vi "quiz3.1.vi"() -> ()   [LabVIEW 2017]
uses:
  <vilib>/Utility/file.llb/Read Delimited Spreadsheet (string).vi
panel:
  out "Tab Control 2":T1(tab)
  in  "Contraseña 2":string
  in  "Login 2":string
  in  "Ingresar 2":bool=TRUE
  in  "Ingrese posicion 2":i32
  in  "Usuario a borrar 2":string
  in  "Agregar 2":bool
  in  "Nuevo usuario 2":string
  in  "Nueva contraseña 2":string
  in  "eliminar 2":bool
  in  "Terminar sesion 3":bool
  out "Usuario 2":string
  in  "Terminar sesion 4":bool
  out "leeradd 2":string[][](array[string])
  out "element 4":string
  out "Usuarios y contraseñas 2":string[](array[string])
  out "element 3":i32
  out "Usuarios 2":string[](array[string])
  out "Usuarios":string[](array[string])
  out "element 2":i32
  out "Usuarios y contraseñas":string[](array[string])
  out "leeradd":string[][](array[string])
  out "element":string
  out "Tab Control":T1(tab)
  in  "Contraseña":string
  in  "Login":string
  in  "Ingresar":bool=TRUE
  in  "Ingrese posicion":i32
  in  "Usuario a borrar":string
  in  "Agregar":bool
  in  "Nuevo usuario":string
  in  "Nueva contraseña":string
  in  "eliminar":bool
  in  "Terminar sesion 2":bool
  out "Usuario":string
  in  "Terminar sesion":bool
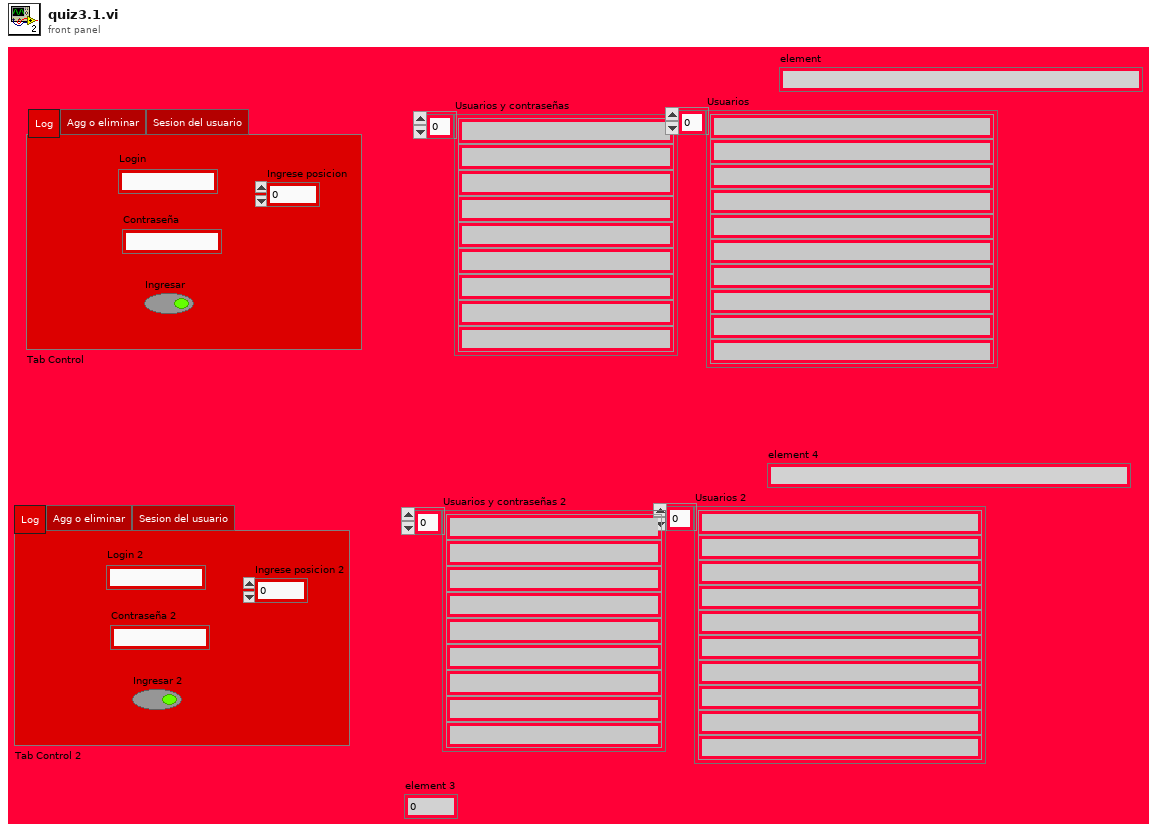
[diagram p1: front panel]
types:
  T1 = enum32{"Log", "Agg o eliminar", "Sesion del usuario"}
  T2 = enum16{"open", "replace", "create", "open or create", "replace or create", "replace or create with confirmation"}
  T3 = typedef "Semaphore RefNum" = refnum<k1>
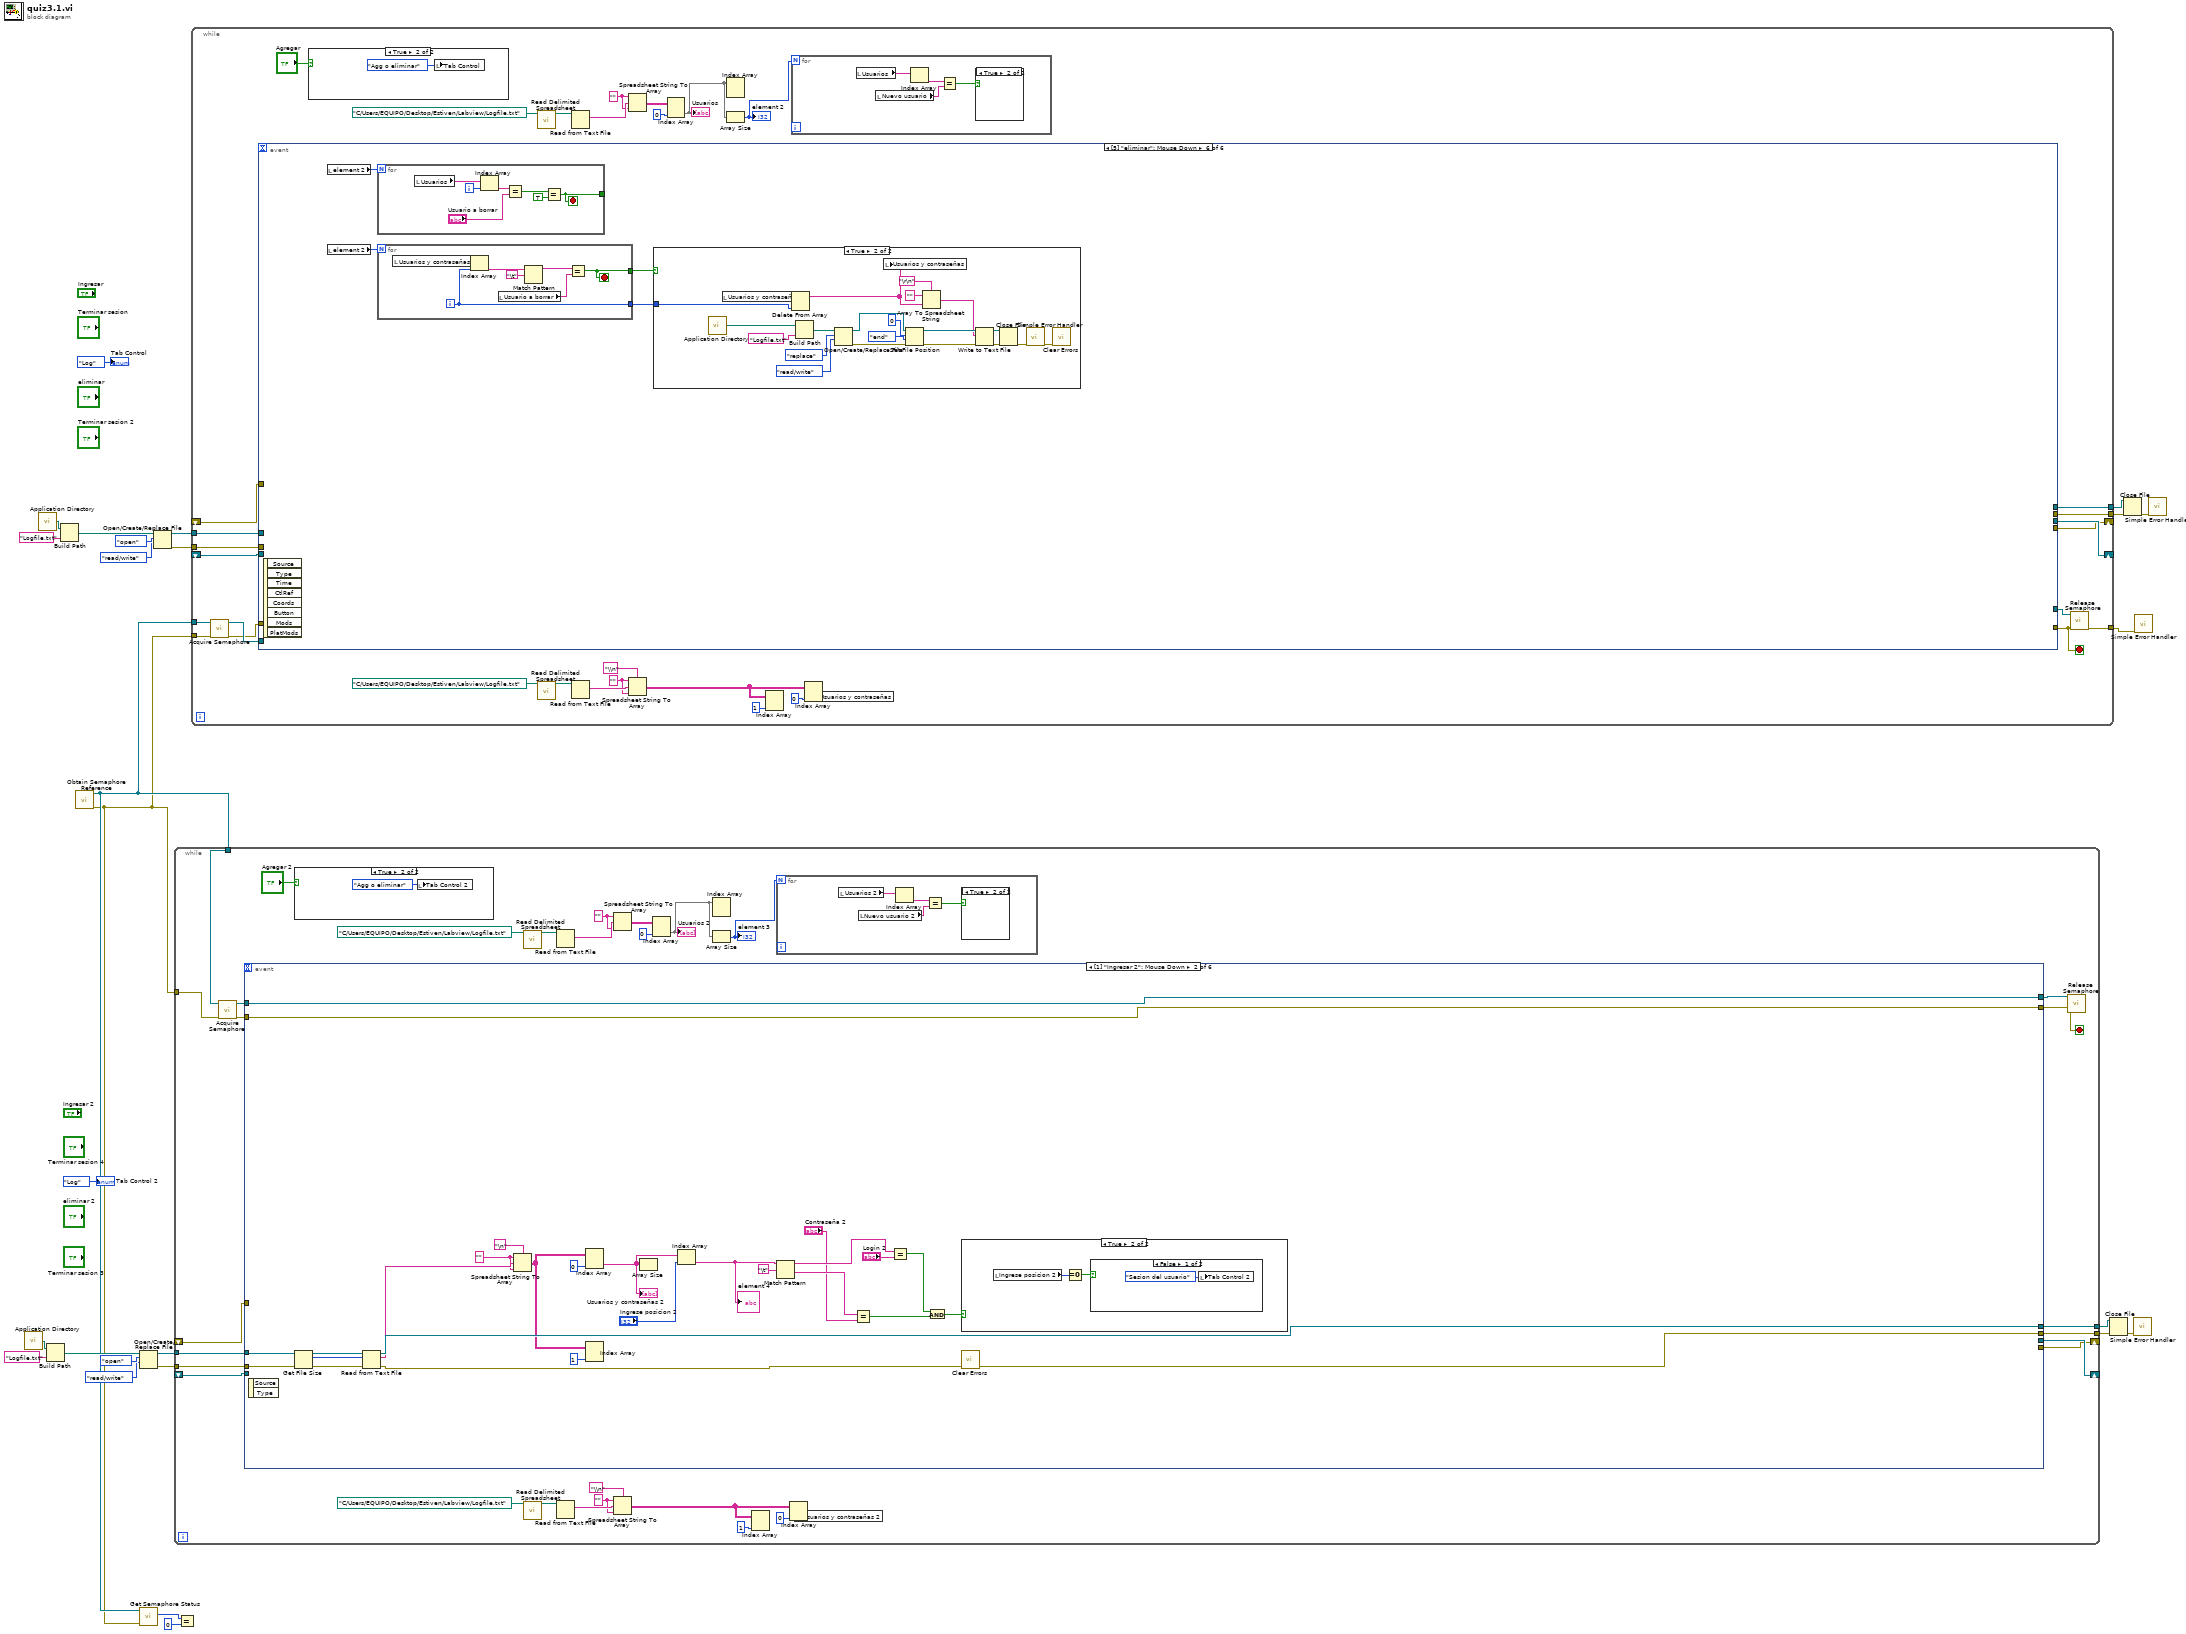
[diagram p0: block diagram]
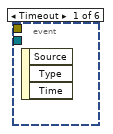
[diagram p4: hidden frame]
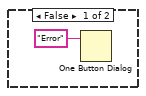
[diagram p5: hidden frame]
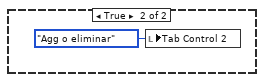
[diagram p6: hidden frame]
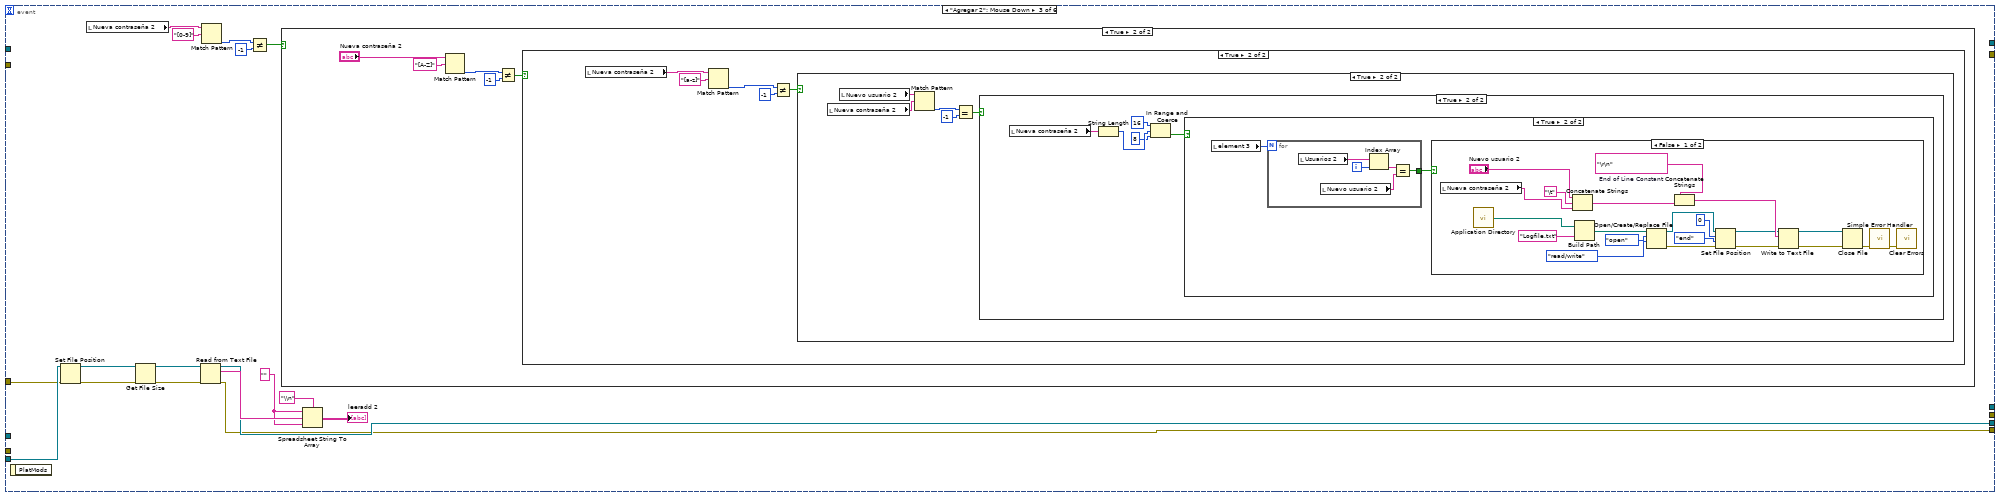
[diagram p7: hidden frame]
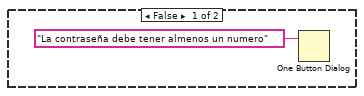
[diagram p8: hidden frame]
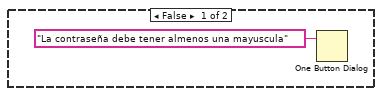
[diagram p9: hidden frame]
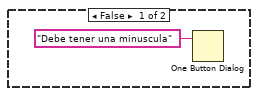
[diagram p10: hidden frame]
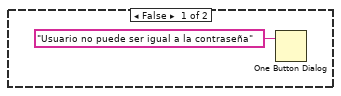
[diagram p11: hidden frame]
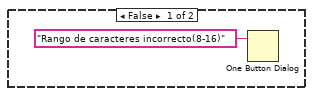
[diagram p12: hidden frame]
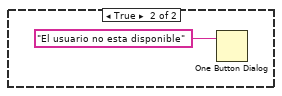
[diagram p13: hidden frame]
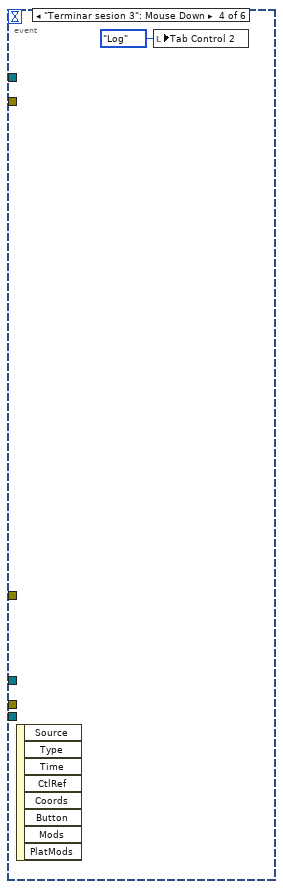
[diagram p14: hidden frame]
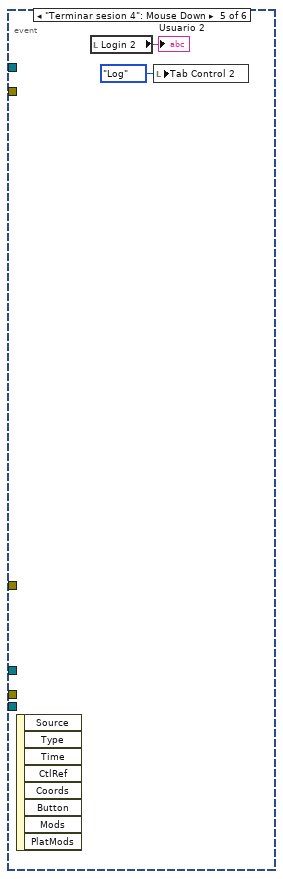
[diagram p15: hidden frame]
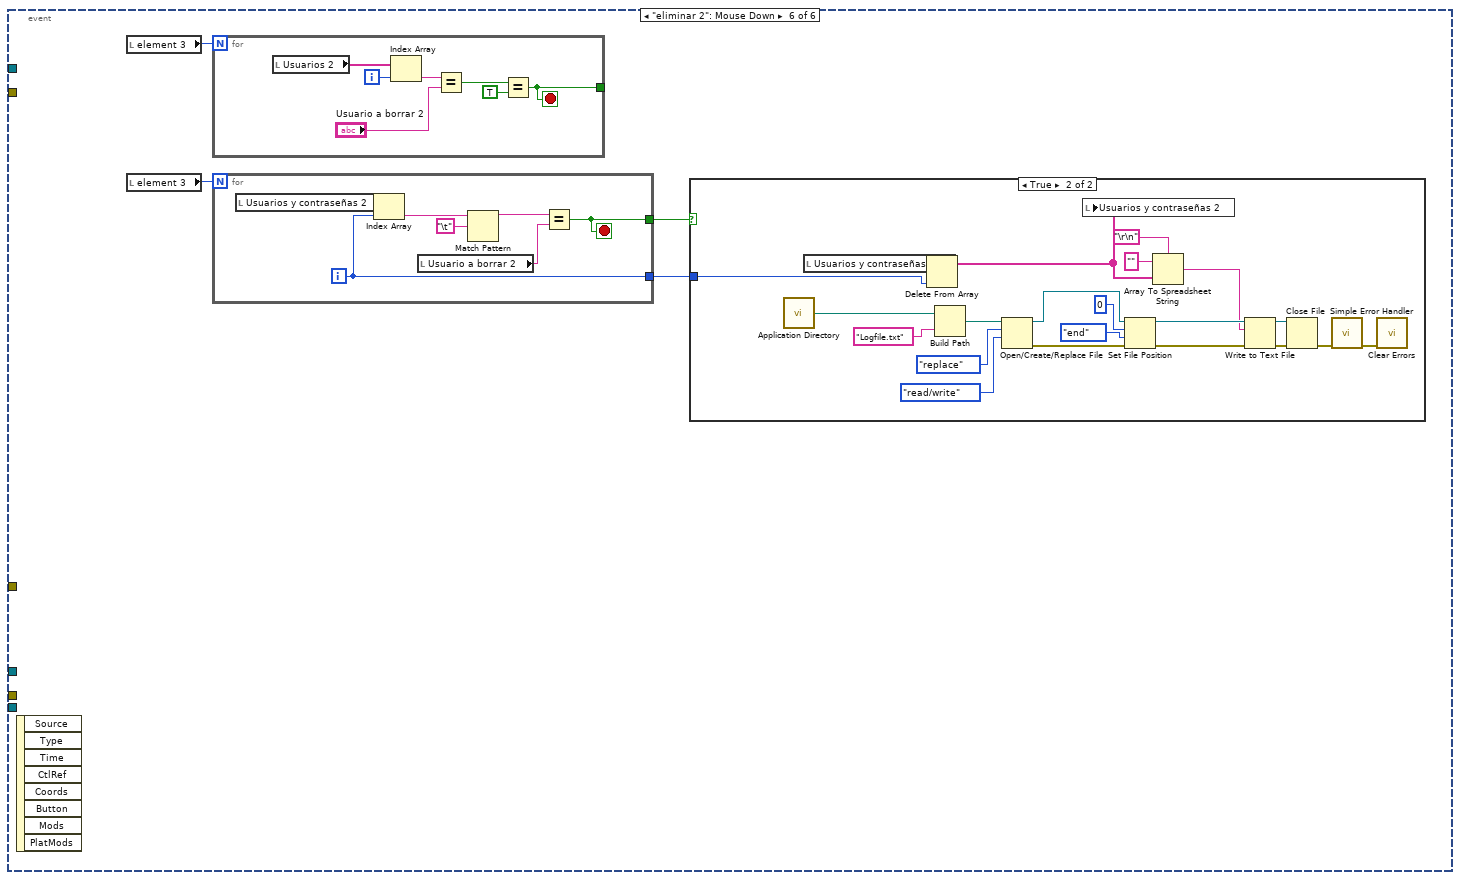
[diagram p16: hidden frame]
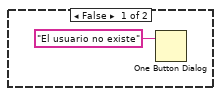
[diagram p17: hidden frame]
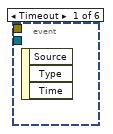
[diagram p20: hidden frame]
diagram:
  n1 = call <vilib>:"Application Directory.vi"() -> ("Application Directory"=w10:path)
  n2 = call <vilib>:"Application Directory.vi"() -> ("Application Directory"=w21:path)
  n3 = Build Path(base path=w10, name or relative path="Logfile.txt") -> (appended path=w11:path)
  n4 = Build Path(base path=w21, name or relative path="Logfile.txt") -> (appended path=w22:path)
  n5 = call <vilib>:"Obtain Semaphore Reference.vi"() -> ("error out"=w3:errorcluster, "semaphore"=w4:T3)  [unwired: 5 in, 1 out]
  n6 = Open/Create/Replace File(file path (use dialog)=w11, operation (0:open)=T2."open", access (0:read/write)=enum16{"read/write", "read-only", "write-only"}."read/write") -> (refnum out=w13:refnum<file>, error out=w16:errorcluster)  [unwired: 3 in, 1 out]
  n7 = call <vilib>:"Get Semaphore Status.vi"("error in (no error)"=w3, "semaphore"=w4) -> ("# available"=w2:i32)  [unwired: 4 in, 5 out]
  n8 = Open/Create/Replace File(file path (use dialog)=w22, operation (0:open)=T2."open", access (0:read/write)=enum16{"read/write", "read-only", "write-only"}."read/write") -> (refnum out=w24:refnum<file>, error out=w27:errorcluster)  [unwired: 3 in, 1 out]
  n9 = while {
    tunnel: w16 -> [w55]
    tunnel: [w59] -> w15
    tunnel: w13 -> [w58]
    tunnel: [w57] -> w12
    shift-right: [w52] -> _
    shift-left: _ -> [w54]
    shift-right: [w51] -> _
    shift-left: _ -> [w53]
    tunnel: w4 -> [w33]
    tunnel: w3 -> [w32]
    stop <- w28 stop-if-true
    w36 = "" ("format string")
    w46 = "" ("format string")
    n10 = call <vilib>:"Acquire Semaphore.vi"("error in (no error)"=w32, "semaphore"=w33) -> ("error out"=w29:errorcluster, "semaphore out"=w31:T3)  [unwired: 3 in, 1 out]
    n11 = event shown="[1] \"Ingresar 2\": Mouse Down" {
      selector: _ -> [_ _ _ _ _ _]
      dyn-events: _ -> [_ _ _ _ _ _]
      timeout: _ -> [_ _ _ _ _ _]
      tunnel: w55 -> [_ w83 _ _ _ _]
      tunnel: [_ w90 _ _ _ _] -> w59
      tunnel: w58 -> [_ w84 _ _ _ _]
      tunnel: [_ w86 _ _ _ _] -> w57
      tunnel: w54 -> [_ _ w101 _ _ _]
      tunnel: w53 -> [_ _ w100 _ _ _]
      tunnel: [_ _ w98 _ _ _] -> w52
      tunnel: [_ _ w97 _ _ _] -> w51
      tunnel: [_ w66 _ _ _ _] -> w30
      tunnel: w31 -> [_ w66 _ _ _ _]
      tunnel: w29 -> [_ w65 _ _ _ _]
      tunnel: [_ w65 _ _ _ _] -> w28
      event Timeout {
        n12 = event-data() -> ()  [unwired: 1 in, 3 out]
      }
      event "Ingresar 2": Mouse Down {
        w76 = "" ("format string")
        n13 = event-data() -> ()  [unwired: 1 in, 2 out]
        n14 = Get File Size(file=w84, error in=w83) -> (refnum out=w82:refnum<file>, size (in bytes)=w81:i64, 0:w80:errorcluster)
        n15 = Read from Text File(file (use dialog)=w82, count=w81, error in=w80) -> (refnum out=w86:refnum<file>, text=w77:string, error out=w91:errorcluster)  [unwired: 1 in, 1 out]
        n16 = Spreadsheet String To Array(delimiter (Tab)="\n", format string=w76, spreadsheet string=w77, array type (2D Dbl)=w76) -> (array=w75:string[][])
        n17 = Index Array "Index Array"(array=w75, index (col)=0 ("disabled index (col)")) -> (element=w67:string[])  [unwired: 1 in]
        "Usuarios y contraseñas 2" <- w67
        n18 = Index Array "Index Array"(array=w75, index (col)=1 ("disabled index (col)")) -> ()  [unwired: 1 in, 1 out]
        n19 = Array Size(array=w67) -> ()  [unwired: 1 out]
        n20 = Index Array "Index Array"(array=w67, index="Ingrese posicion 2") -> (element=w68:string)
        "element 4" <- w68
        n21 = Match Pattern(string=w68, regular expression="\t") -> (before substring=w79:string, after substring=w78:string)  [unwired: 1 in, 2 out]
        n22 = Equal?(x=w78, y="Contraseña 2") -> (x = y?=w88:bool)
        n23 = Equal?(x=w79, y="Login 2") -> (x = y?=w89:bool)
        n24 = And(x=w89, y=w88) -> (x .and. y?=w87:bool)
        n25 = case shown="True" w87 {
          frame False {
            n26 = One Button Dialog(message="Error") -> ()  [unwired: 1 in, 1 out]
          }
          frame True {
            n27 = local read "Ingrese posicion 2"() -> (w94:i32)
            n28 = Equal To 0?(x=w94) -> (x = 0?=w93:bool)
            n29 = case shown="False" w93 {
              frame False {
                n30 = local write "Tab Control 2"(T1."Sesion del usuario" ("Tab Control")) -> ()
              }
              frame True {
                n31 = local write "Tab Control 2"(enum32{"Log", "Agg o eliminar"}."Agg o eliminar" ("Tab Control")) -> ()
              }
            }
          }
        }
        n32 = call <vilib>:"Clear Errors.vi"("error in (no error)"=w91) -> ("error out"=w90:errorcluster)  [unwired: 5 in, 1 out]
      }
      event "Agregar 2": Mouse Down {
        w102 = "" ("format string")
        n33 = event-data() -> ()  [unwired: 1 in, 1 out]
        n34 = Set File Position(refnum=w101, error in=w100) -> (refnum out=w108:refnum<file>, error out=w105:errorcluster)  [unwired: 2 in]
        n35 = local read "Nueva contraseña 2"() -> (w113:string)
        n36 = Get File Size(file=w108, error in=w105) -> (refnum out=w107:refnum<file>, 0:w104:errorcluster)  [unwired: 1 out]
        n37 = Read from Text File(file (use dialog)=w107, error in=w104) -> (refnum out=w98:refnum<file>, text=w106:string, error out=w97:errorcluster)  [unwired: 2 in, 1 out]
        n38 = Match Pattern(string=w113, regular expression="[0-9]") -> (offset past match=w111:i32)  [unwired: 1 in, 3 out]
        n39 = Not Equal?(x=w111, y=-1) -> (x != y?=w109:bool)
        n40 = case shown="True" w109 {
          frame False {
            n41 = One Button Dialog(message="La contraseña debe tener almenos un numero") -> ()  [unwired: 1 in, 1 out]
          }
          frame True {
            n42 = Match Pattern(string="Nueva contraseña 2", regular expression="[A-Z]") -> (offset past match=w118:i32)  [unwired: 1 in, 3 out]
            n43 = Not Equal?(x=w118, y=-1) -> (x != y?=w115:bool)
            n44 = case shown="True" w115 {
              frame False {
                n45 = One Button Dialog(message="La contraseña debe tener almenos una mayuscula") -> ()  [unwired: 1 in, 1 out]
              }
              frame True {
                n46 = local read "Nueva contraseña 2"() -> (w122:string)
                n47 = Match Pattern(string=w122, regular expression="[a-z]") -> (offset past match=w124:i32)  [unwired: 1 in, 3 out]
                n48 = Not Equal?(x=w124, y=-1) -> (x != y?=w121:bool)
                n49 = case shown="True" w121 {
                  frame False {
                    n50 = One Button Dialog(message="Debe tener una minuscula") -> ()  [unwired: 1 in, 1 out]
                  }
                  frame True {
                    n51 = local read "Nueva contraseña 2"() -> (w131:string)
                    n52 = local read "Nuevo usuario 2"() -> (w130:string)
                    n53 = Match Pattern(string=w130, regular expression=w131) -> (offset past match=w129:i32)  [unwired: 1 in, 3 out]
                    n54 = Equal?(x=w129, y=-1) -> (x = y?=w128:bool)
                    n55 = case shown="True" w128 {
                      frame False {
                        n56 = One Button Dialog(message="Usuario no puede ser igual a la contraseña") -> ()  [unwired: 1 in, 1 out]
                      }
                      frame True {
                        n57 = local read "Nueva contraseña 2"() -> (w137:string)
                        n58 = String Length(string=w137) -> (length=w136:i32)
                        n59 = In Range and Coerce(upper limit=16, x=w136, lower limit=8) -> (In Range?=w133:bool)  [unwired: 1 out]
                        n60 = case shown="True" w133 {
                          frame False {
                            n61 = One Button Dialog(message="Rango de caracteres incorrecto(8-16)") -> ()  [unwired: 1 in, 1 out]
                          }
                          frame True {
                            n62 = local read "element 3"() -> (w140:i32)
                            n63 = for {
                              N: w140 -> [_]
                              tunnel: [w165] -> w139
                              i -> [w163]
                              n64 = local read "Usuarios 2"() -> (w164:string[])
                              n65 = local read "Nuevo usuario 2"() -> (w167:string)
                              n66 = Index Array(array=w164, index=w163) -> (element=w166:string)
                              n67 = Equal?(x=w166, y=w167) -> (x = y?=w165:bool)
                            }
                            n68 = case shown="False" w139 {
                              frame False {
                                w147 = "\r\n"  # End of Line Constant
                                n69 = local read "Nueva contraseña 2"() -> (w148:string)
                                n70 = call <vilib>:"Application Directory.vi"() -> ("Application Directory"=w150:path)
                                n71 = Concatenate Strings "Concatenate Strings"("Nuevo usuario 2", "\t", w148) -> (w161:string)
                                n72 = Build Path(base path=w150, name or relative path="Logfile.txt") -> (appended path=w151:path)
                                n73 = Open/Create/Replace File(file path (use dialog)=w151, operation (0:open)=T2."open", access (0:read/write)=enum16{"read/write", "read-only", "write-only"}."read/write") -> (refnum out=w152:refnum<file>, error out=w155:errorcluster)  [unwired: 3 in, 1 out]
                                n74 = Concatenate Strings "Concatenate Strings"(w147, w161) -> (w160:string)
                                n75 = Set File Position(offset (in bytes) (0)=i64 0, refnum=w152, from (0:start)=enum16{"start", "end", "current"}."end", error in=w155) -> (refnum out=w153:refnum<file>, error out=w156:errorcluster)
                                n76 = Write to Text File(file (use dialog)=w153, text=w160, error in=w156) -> (refnum out=w154:refnum<file>, error out=w157:errorcluster)  [unwired: 1 in, 1 out]
                                n77 = Close File(refnum=w154, error in=w157) -> (error out=w158:errorcluster)  [unwired: 1 out]
                                n78 = call <vilib>:"Simple Error Handler.vi"("error in (no error)"=w158) -> ("error out"=w159:errorcluster)  [unwired: 4 in, 4 out]
                                n79 = call <vilib>:"Clear Errors.vi"("error in (no error)"=w159) -> ()  [unwired: 5 in, 2 out]
                              }
                              frame True {
                                n80 = One Button Dialog(message="El usuario no esta disponible") -> ()  [unwired: 1 in, 1 out]
                              }
                            }
                          }
                        }
                      }
                    }
                  }
                }
              }
            }
          }
        }
        n81 = Spreadsheet String To Array(delimiter (Tab)="\\n", format string=w102, spreadsheet string=w106, array type (2D Dbl)=w102) -> (array=→"leeradd 2":string[][])
      }
      event "Terminar sesion 3": Mouse Down {
        n82 = event-data() -> ()  [unwired: 1 in, 8 out]
        n83 = local write "Tab Control 2"(T1."Log" ("Tab Control")) -> ()
      }
      event "Terminar sesion 4": Mouse Down {
        n84 = event-data() -> ()  [unwired: 1 in, 8 out]
        n85 = local read "Login 2"() -> (→"Usuario 2":string)
        n86 = local write "Tab Control 2"(T1."Log" ("Tab Control")) -> ()
      }
      event "eliminar 2": Mouse Down {
        n87 = event-data() -> ()  [unwired: 1 in, 8 out]
        n88 = local read "element 3"() -> (w174:i32)
        n89 = local read "element 3"() -> (w173:i32)
        n90 = for {
          N: w174 -> [_]
          tunnel: [w183] -> _
          i -> [w182]
          stop <- w183 stop-if-true
          n91 = local read "Usuarios 2"() -> (w185:string[])
          n92 = Index Array(array=w185, index=w182) -> (element=w184:string)
          n93 = Equal?(x=w184, y="Usuario a borrar 2") -> (x = y?=w188:bool)
          n94 = Equal?(x=w188, y=TRUE) -> (x = y?=w183:bool)
        }
        n95 = for {
          N: w173 -> [_]
          tunnel: [w177] -> w171
          tunnel: [w175] -> w172
          i -> [w175]
          stop <- w177 stop-if-true
          n96 = local read "Usuarios y contraseñas 2"() -> (w176:string[])
          n97 = Index Array(array=w176, index=w175) -> (element=w181:string)
          n98 = local read "Usuario a borrar 2"() -> (w178:string)
          n99 = Match Pattern(string=w181, regular expression="\t") -> (before substring=w179:string)  [unwired: 1 in, 3 out]
          n100 = Equal?(x=w179, y=w178) -> (x = y?=w177:bool)
        }
        n101 = case shown="True" w171 {
          tunnel: w172 -> [_ w195]
          frame False {
            n102 = One Button Dialog(message="El usuario no existe") -> ()  [unwired: 1 in, 1 out]
          }
          frame True {
            n103 = call <vilib>:"Application Directory.vi"() -> ("Application Directory"=w201:path)
            n104 = local read "Usuarios y contraseñas 2"() -> (w194:string[])
            n105 = Delete From Array "Delete From Array"(array=w194, index=w195) -> (array with subset deleted=w192:string[])  [unwired: 1 in, 1 out]
            n106 = Build Path(base path=w201, name or relative path="Logfile.txt") -> (appended path=w202:path)
            n107 = Open/Create/Replace File(file path (use dialog)=w202, operation (0:open)=T2."replace", access (0:read/write)=enum16{"read/write", "read-only", "write-only"}."read/write") -> (refnum out=w203:refnum<file>, error out=w206:errorcluster)  [unwired: 3 in, 1 out]
            n108 = local write "Usuarios y contraseñas 2"(w192) -> ()
            n109 = Set File Position(offset (in bytes) (0)=i64 0, refnum=w203, from (0:start)=enum16{"start", "end", "current"}."end", error in=w206) -> (refnum out=w204:refnum<file>, error out=w207:errorcluster)
            n110 = Array To Spreadsheet String(delimiter (Tab)="\r\n", array=w192, 3:"" ("format string")) -> (spreadsheet string=w191:string)
            n111 = Write to Text File(file (use dialog)=w204, text=w191, error in=w207) -> (refnum out=w205:refnum<file>, error out=w208:errorcluster)  [unwired: 1 in, 1 out]
            n112 = Close File(refnum=w205, error in=w208) -> (error out=w209:errorcluster)  [unwired: 1 out]
            n113 = call <vilib>:"Simple Error Handler.vi"("error in (no error)"=w209) -> ("error out"=w210:errorcluster)  [unwired: 4 in, 4 out]
            n114 = call <vilib>:"Clear Errors.vi"("error in (no error)"=w210) -> ()  [unwired: 5 in, 2 out]
          }
        }
      }
    }
    n115 = case shown="True" "Agregar 2" {
      frame False {
      }
      frame True {
        n116 = local write "Tab Control 2"(T1."Agg o eliminar" ("Tab Control")) -> ()
      }
    }
    n117 = call-poly <vilib>:"Read Delimited Spreadsheet.vi"("file path (dialog if empty)"=path "C:/Users/EQUIPO/Desktop/Estiven/Labview/Logfile.txt") -> ("new file path (Not A Path if cancelled)"=w47:path)  [unwired: 9 in, 5 out]
    n118 = call-poly <vilib>:"Read Delimited Spreadsheet.vi"("file path (dialog if empty)"=path "C:/Users/EQUIPO/Desktop/Estiven/Labview/Logfile.txt") -> ("new file path (Not A Path if cancelled)"=w42:path)  [unwired: 9 in, 5 out]
    n119 = Read from Text File(file (use dialog)=w47) -> (text=w48:string)  [unwired: 3 in, 3 out]
    n120 = Read from Text File(file (use dialog)=w42) -> (text=w41:string)  [unwired: 3 in, 3 out]
    n121 = Spreadsheet String To Array(format string=w46, spreadsheet string=w48, array type (2D Dbl)=w46) -> (array=w49:string[][])  [unwired: 1 in]
    n122 = Spreadsheet String To Array(delimiter (Tab)="\\n", format string=w36, spreadsheet string=w41, array type (2D Dbl)=w36) -> (array=w40:string[][])
    n123 = Index Array(array=w49, index (col)=0 ("index")) -> (element=w43:string[])  [unwired: 1 in]
    "Usuarios 2" <- w43
    n124 = Index Array "Index Array"(array=w43) -> ()  [unwired: 2 in, 2 out]
    n125 = Array Size(array=w43) -> (size(s)=w50:i32)
    "element 3" <- w50
    n126 = Index Array(array=w40, index (col)=1 ("disabled index (col)")) -> ()  [unwired: 1 in, 1 out]
    n127 = for {
      N: w50 -> [_]
      n128 = local read "Usuarios 2"() -> (w63:string[])
      n129 = local read "Nuevo usuario 2"() -> (w61:string)
      n130 = Index Array(array=w63) -> (element=w62:string)  [unwired: 1 in]
      n131 = Equal?(x=w62, y=w61) -> (x = y?=w60:bool)
      n132 = case shown="True" w60 {
        frame False {
        }
        frame True {
        }
      }
    }
    n133 = Index Array(array=w40, index (col)=0 ("index")) -> (element=w39:string[])  [unwired: 1 in]
    n134 = local write "Usuarios y contraseñas 2"(w39) -> ()
    n135 = call <vilib>:"Release Semaphore.vi"("error in (no error)"=w28, "semaphore"=w30) -> ()  [unwired: 4 in, 2 out]
  }
  n136 = Equal?(x=w2, y=0) -> ()  [unwired: 1 out]
  n137 = while {
    tunnel: w27 -> [w239]
    tunnel: [w243] -> w26
    tunnel: w24 -> [w242]
    tunnel: [w241] -> w23
    shift-right: [w236] -> _
    shift-left: _ -> [w238]
    shift-right: [w235] -> _
    shift-left: _ -> [w237]
    tunnel: w4 -> [w217]
    tunnel: w3 -> [w216]
    tunnel: [w211] -> w5
    stop <- w212 stop-if-true
    w220 = "" ("format string")
    w230 = "" ("format string")
    n138 = call <vilib>:"Acquire Semaphore.vi"("error in (no error)"=w216, "semaphore"=w217) -> ("error out"=w213:errorcluster, "semaphore out"=w215:T3)  [unwired: 3 in, 1 out]
    n139 = event shown="[5] \"eliminar\": Mouse Down" {
      selector: _ -> [_ _ _ _ _ _]
      dyn-events: _ -> [_ _ _ _ _ _]
      timeout: _ -> [_ _ _ _ _ _]
      tunnel: w239 -> [_ w267 _ _ _ _]
      tunnel: [_ w274 _ _ _ _] -> w243
      tunnel: w242 -> [_ w268 _ _ _ _]
      tunnel: [_ w270 _ _ _ _] -> w241
      tunnel: w238 -> [_ _ w286 _ _ _]
      tunnel: w237 -> [_ _ w285 _ _ _]
      tunnel: [_ _ w283 _ _ _] -> w236
      tunnel: [_ _ w282 _ _ _] -> w235
      tunnel: [_ w250 _ _ _ _] -> w214
      tunnel: w215 -> [_ w250 _ _ _ _]
      tunnel: w213 -> [_ w249 _ _ _ _]
      tunnel: [_ w249 _ _ _ _] -> w212
      event Timeout {
        n140 = event-data() -> ()  [unwired: 1 in, 3 out]
      }
      event "Ingresar": Mouse Down {
        w260 = "" ("format string")
        n141 = event-data() -> ()  [unwired: 1 in, 2 out]
        n142 = Get File Size(file=w268, error in=w267) -> (refnum out=w266:refnum<file>, size (in bytes)=w265:i64, 0:w264:errorcluster)
        n143 = Read from Text File(file (use dialog)=w266, count=w265, error in=w264) -> (refnum out=w270:refnum<file>, text=w261:string, error out=w275:errorcluster)  [unwired: 1 in, 1 out]
        n144 = Spreadsheet String To Array(delimiter (Tab)="\n", format string=w260, spreadsheet string=w261, array type (2D Dbl)=w260) -> (array=w259:string[][])
        n145 = Index Array "Index Array"(array=w259, index (col)=0 ("disabled index (col)")) -> (element=w251:string[])  [unwired: 1 in]
        "Usuarios y contraseñas" <- w251
        n146 = Index Array "Index Array"(array=w259, index (col)=1 ("disabled index (col)")) -> ()  [unwired: 1 in, 1 out]
        n147 = Array Size(array=w251) -> ()  [unwired: 1 out]
        n148 = Index Array "Index Array"(array=w251, index="Ingrese posicion") -> (element=w252:string)
        "element" <- w252
        n149 = Match Pattern(string=w252, regular expression="\t") -> (before substring=w263:string, after substring=w262:string)  [unwired: 1 in, 2 out]
        n150 = Equal?(x=w262, y="Contraseña") -> (x = y?=w272:bool)
        n151 = Equal?(x=w263, y="Login") -> (x = y?=w273:bool)
        n152 = And(x=w273, y=w272) -> (x .and. y?=w271:bool)
        n153 = case shown="True" w271 {
          frame False {
            n154 = One Button Dialog(message="Error") -> ()  [unwired: 1 in, 1 out]
          }
          frame True {
            n155 = local read "Ingrese posicion"() -> (w278:i32)
            n156 = Equal To 0?(x=w278) -> (x = 0?=w277:bool)
            n157 = case shown="False" w277 {
              frame False {
                n158 = local read "Login"() -> (→"Usuario":string)
                n159 = local write "Tab Control"(T1."Sesion del usuario" ("Tab Control")) -> ()
              }
              frame True {
                n160 = local write "Tab Control"(enum32{"Log", "Agg o eliminar"}."Agg o eliminar" ("Tab Control")) -> ()
              }
            }
          }
        }
        n161 = call <vilib>:"Clear Errors.vi"("error in (no error)"=w275) -> ("error out"=w274:errorcluster)  [unwired: 5 in, 1 out]
      }
      event "Agregar": Mouse Down {
        w287 = "" ("format string")
        n162 = event-data() -> ()  [unwired: 1 in, 1 out]
        n163 = Set File Position(refnum=w286, error in=w285) -> (refnum out=w293:refnum<file>, error out=w290:errorcluster)  [unwired: 2 in]
        n164 = local read "Nueva contraseña"() -> (w298:string)
        n165 = Get File Size(file=w293, error in=w290) -> (refnum out=w292:refnum<file>, 0:w289:errorcluster)  [unwired: 1 out]
        n166 = Read from Text File(file (use dialog)=w292, error in=w289) -> (refnum out=w283:refnum<file>, text=w291:string, error out=w282:errorcluster)  [unwired: 2 in, 1 out]
        n167 = Match Pattern(string=w298, regular expression="[0-9]") -> (offset past match=w296:i32)  [unwired: 1 in, 3 out]
        n168 = Not Equal?(x=w296, y=-1) -> (x != y?=w294:bool)
        n169 = case shown="True" w294 {
          frame False {
            n170 = One Button Dialog(message="La contraseña debe tener almenos un numero") -> ()  [unwired: 1 in, 1 out]
          }
          frame True {
            n171 = Match Pattern(string="Nueva contraseña", regular expression="[A-Z]") -> (offset past match=w303:i32)  [unwired: 1 in, 3 out]
            n172 = Not Equal?(x=w303, y=-1) -> (x != y?=w300:bool)
            n173 = case shown="True" w300 {
              frame False {
                n174 = One Button Dialog(message="La contraseña debe tener almenos una mayuscula") -> ()  [unwired: 1 in, 1 out]
              }
              frame True {
                n175 = local read "Nueva contraseña"() -> (w307:string)
                n176 = Match Pattern(string=w307, regular expression="[a-z]") -> (offset past match=w309:i32)  [unwired: 1 in, 3 out]
                n177 = Not Equal?(x=w309, y=-1) -> (x != y?=w306:bool)
                n178 = case shown="True" w306 {
                  frame False {
                    n179 = One Button Dialog(message="Debe tener una minuscula") -> ()  [unwired: 1 in, 1 out]
                  }
                  frame True {
                    n180 = local read "Nueva contraseña"() -> (w316:string)
                    n181 = local read "Nuevo usuario"() -> (w315:string)
                    n182 = Match Pattern(string=w315, regular expression=w316) -> (offset past match=w314:i32)  [unwired: 1 in, 3 out]
                    n183 = Equal?(x=w314, y=-1) -> (x = y?=w313:bool)
                    n184 = case shown="True" w313 {
                      frame False {
                        n185 = One Button Dialog(message="Usuario no puede ser igual a la contraseña") -> ()  [unwired: 1 in, 1 out]
                      }
                      frame True {
                        n186 = local read "Nueva contraseña"() -> (w322:string)
                        n187 = String Length(string=w322) -> (length=w321:i32)
                        n188 = In Range and Coerce(upper limit=16, x=w321, lower limit=8) -> (In Range?=w318:bool)  [unwired: 1 out]
                        n189 = case shown="True" w318 {
                          frame False {
                            n190 = One Button Dialog(message="Rango de caracteres incorrecto(8-16)") -> ()  [unwired: 1 in, 1 out]
                          }
                          frame True {
                            n191 = local read "element 2"() -> (w325:i32)
                            n192 = for {
                              N: w325 -> [_]
                              tunnel: [w350] -> w324
                              i -> [w348]
                              n193 = local read "Usuarios"() -> (w349:string[])
                              n194 = local read "Nuevo usuario"() -> (w352:string)
                              n195 = Index Array(array=w349, index=w348) -> (element=w351:string)
                              n196 = Equal?(x=w351, y=w352) -> (x = y?=w350:bool)
                            }
                            n197 = case shown="False" w324 {
                              frame False {
                                w332 = "\r\n"  # End of Line Constant
                                n198 = local read "Nueva contraseña"() -> (w333:string)
                                n199 = call <vilib>:"Application Directory.vi"() -> ("Application Directory"=w335:path)
                                n200 = Concatenate Strings "Concatenate Strings"("Nuevo usuario", "\t", w333) -> (w346:string)
                                n201 = Build Path(base path=w335, name or relative path="Logfile.txt") -> (appended path=w336:path)
                                n202 = Open/Create/Replace File(file path (use dialog)=w336, operation (0:open)=T2."open", access (0:read/write)=enum16{"read/write", "read-only", "write-only"}."read/write") -> (refnum out=w337:refnum<file>, error out=w340:errorcluster)  [unwired: 3 in, 1 out]
                                n203 = Concatenate Strings "Concatenate Strings"(w332, w346) -> (w345:string)
                                n204 = Set File Position(offset (in bytes) (0)=i64 0, refnum=w337, from (0:start)=enum16{"start", "end", "current"}."end", error in=w340) -> (refnum out=w338:refnum<file>, error out=w341:errorcluster)
                                n205 = Write to Text File(file (use dialog)=w338, text=w345, error in=w341) -> (refnum out=w339:refnum<file>, error out=w342:errorcluster)  [unwired: 1 in, 1 out]
                                n206 = Close File(refnum=w339, error in=w342) -> (error out=w343:errorcluster)  [unwired: 1 out]
                                n207 = call <vilib>:"Simple Error Handler.vi"("error in (no error)"=w343) -> ("error out"=w344:errorcluster)  [unwired: 4 in, 4 out]
                                n208 = call <vilib>:"Clear Errors.vi"("error in (no error)"=w344) -> ()  [unwired: 5 in, 2 out]
                              }
                              frame True {
                                n209 = One Button Dialog(message="El usuario no esta disponible") -> ()  [unwired: 1 in, 1 out]
                              }
                            }
                          }
                        }
                      }
                    }
                  }
                }
              }
            }
          }
        }
        n210 = Spreadsheet String To Array(delimiter (Tab)="\\n", format string=w287, spreadsheet string=w291, array type (2D Dbl)=w287) -> (array=→"leeradd":string[][])
      }
      event "Terminar sesion 2": Mouse Down {
        n211 = event-data() -> ()  [unwired: 1 in, 8 out]
        n212 = local write "Tab Control"(T1."Log" ("Tab Control")) -> ()
      }
      event "Terminar sesion": Mouse Down {
        n213 = event-data() -> ()  [unwired: 1 in, 8 out]
        n214 = local write "Tab Control"(T1."Log" ("Tab Control")) -> ()
      }
      event "eliminar": Mouse Down {
        n215 = event-data() -> ()  [unwired: 1 in, 8 out]
        n216 = local read "element 2"() -> (w358:i32)
        n217 = local read "element 2"() -> (w357:i32)
        n218 = for {
          N: w358 -> [_]
          tunnel: [w367] -> _
          i -> [w366]
          stop <- w367 stop-if-true
          n219 = local read "Usuarios"() -> (w369:string[])
          n220 = Index Array(array=w369, index=w366) -> (element=w368:string)
          n221 = Equal?(x=w368, y="Usuario a borrar") -> (x = y?=w372:bool)
          n222 = Equal?(x=w372, y=TRUE) -> (x = y?=w367:bool)
        }
        n223 = for {
          N: w357 -> [_]
          tunnel: [w361] -> w355
          tunnel: [w359] -> w356
          i -> [w359]
          stop <- w361 stop-if-true
          n224 = local read "Usuarios y contraseñas"() -> (w360:string[])
          n225 = Index Array(array=w360, index=w359) -> (element=w365:string)
          n226 = local read "Usuario a borrar"() -> (w362:string)
          n227 = Match Pattern(string=w365, regular expression="\t") -> (before substring=w363:string)  [unwired: 1 in, 3 out]
          n228 = Equal?(x=w363, y=w362) -> (x = y?=w361:bool)
        }
        n229 = case shown="True" w355 {
          tunnel: w356 -> [_ w379]
          frame False {
            n230 = One Button Dialog(message="El usuario no existe") -> ()  [unwired: 1 in, 1 out]
          }
          frame True {
            n231 = call <vilib>:"Application Directory.vi"() -> ("Application Directory"=w385:path)
            n232 = local read "Usuarios y contraseñas"() -> (w378:string[])
            n233 = Delete From Array "Delete From Array"(array=w378, index=w379) -> (array with subset deleted=w376:string[])  [unwired: 1 in, 1 out]
            n234 = Build Path(base path=w385, name or relative path="Logfile.txt") -> (appended path=w386:path)
            n235 = Open/Create/Replace File(file path (use dialog)=w386, operation (0:open)=T2."replace", access (0:read/write)=enum16{"read/write", "read-only", "write-only"}."read/write") -> (refnum out=w387:refnum<file>, error out=w390:errorcluster)  [unwired: 3 in, 1 out]
            n236 = local write "Usuarios y contraseñas"(w376) -> ()
            n237 = Set File Position(offset (in bytes) (0)=i64 0, refnum=w387, from (0:start)=enum16{"start", "end", "current"}."end", error in=w390) -> (refnum out=w388:refnum<file>, error out=w391:errorcluster)
            n238 = Array To Spreadsheet String(delimiter (Tab)="\r\n", array=w376, 3:"" ("format string")) -> (spreadsheet string=w375:string)
            n239 = Write to Text File(file (use dialog)=w388, text=w375, error in=w391) -> (refnum out=w389:refnum<file>, error out=w392:errorcluster)  [unwired: 1 in, 1 out]
            n240 = Close File(refnum=w389, error in=w392) -> (error out=w393:errorcluster)  [unwired: 1 out]
            n241 = call <vilib>:"Simple Error Handler.vi"("error in (no error)"=w393) -> ("error out"=w394:errorcluster)  [unwired: 4 in, 4 out]
            n242 = call <vilib>:"Clear Errors.vi"("error in (no error)"=w394) -> ()  [unwired: 5 in, 2 out]
          }
        }
      }
    }
    n243 = case shown="True" "Agregar" {
      frame False {
      }
      frame True {
        n244 = local write "Tab Control"(T1."Agg o eliminar" ("Tab Control")) -> ()
      }
    }
    n245 = call-poly <vilib>:"Read Delimited Spreadsheet.vi"("file path (dialog if empty)"=path "C:/Users/EQUIPO/Desktop/Estiven/Labview/Logfile.txt") -> ("new file path (Not A Path if cancelled)"=w231:path)  [unwired: 9 in, 5 out]
    n246 = call-poly <vilib>:"Read Delimited Spreadsheet.vi"("file path (dialog if empty)"=path "C:/Users/EQUIPO/Desktop/Estiven/Labview/Logfile.txt") -> ("new file path (Not A Path if cancelled)"=w226:path)  [unwired: 9 in, 5 out]
    n247 = Read from Text File(file (use dialog)=w231) -> (text=w232:string)  [unwired: 3 in, 3 out]
    n248 = Read from Text File(file (use dialog)=w226) -> (text=w225:string)  [unwired: 3 in, 3 out]
    n249 = Spreadsheet String To Array(format string=w230, spreadsheet string=w232, array type (2D Dbl)=w230) -> (array=w233:string[][])  [unwired: 1 in]
    n250 = Spreadsheet String To Array(delimiter (Tab)="\\n", format string=w220, spreadsheet string=w225, array type (2D Dbl)=w220) -> (array=w224:string[][])
    n251 = Index Array(array=w233, index (col)=0 ("index")) -> (element=w227:string[])  [unwired: 1 in]
    "Usuarios" <- w227
    n252 = Index Array "Index Array"(array=w227) -> ()  [unwired: 2 in, 2 out]
    n253 = Array Size(array=w227) -> (size(s)=w234:i32)
    "element 2" <- w234
    n254 = Index Array(array=w224, index (col)=1 ("disabled index (col)")) -> ()  [unwired: 1 in, 1 out]
    n255 = for {
      N: w234 -> [_]
      n256 = local read "Usuarios"() -> (w247:string[])
      n257 = local read "Nuevo usuario"() -> (w245:string)
      n258 = Index Array(array=w247) -> (element=w246:string)  [unwired: 1 in]
      n259 = Equal?(x=w246, y=w245) -> (x = y?=w244:bool)
      n260 = case shown="True" w244 {
        frame False {
        }
        frame True {
        }
      }
    }
    n261 = Index Array(array=w224, index (col)=0 ("index")) -> (element=w223:string[])  [unwired: 1 in]
    n262 = local write "Usuarios y contraseñas"(w223) -> ()
    n263 = call <vilib>:"Release Semaphore.vi"("error in (no error)"=w212, "semaphore"=w214) -> ("error out"=w211:errorcluster)  [unwired: 4 in, 1 out]
  }
  n264 = Close File(refnum=w12, error in=w15) -> (error out=w14:errorcluster)  [unwired: 1 out]
  n265 = Close File(refnum=w23, error in=w26) -> (error out=w25:errorcluster)  [unwired: 1 out]
  n266 = call <vilib>:"Simple Error Handler.vi"("error in (no error)"=w14) -> ()  [unwired: 4 in, 5 out]
  n267 = call <vilib>:"Simple Error Handler.vi"("error in (no error)"=w5) -> ()  [unwired: 4 in, 5 out]
  n268 = call <vilib>:"Simple Error Handler.vi"("error in (no error)"=w25) -> ()  [unwired: 4 in, 5 out]
  "Tab Control" <- T1."Log" ("Tab Control")
  "Tab Control 2" <- T1."Log" ("Tab Control")
